vi "Get Pending IMatch Responses.vi"(8 "error in":errorcluster, 11 "Response Matcher in":refnum<class "Response Matcher.lvclass">) -> (0 "error out":errorcluster, 2 "Pending IMatch Responses":refnum<data-value>, 3 "Response Matcher out":refnum<class "Response Matcher.lvclass">)   [LabVIEW 2020, in "CANopen.lvlib" / "Response Matcher.lvlib" / "Response Matcher.lvclass"]
uses:
  Response Matcher.lvclass
  IResponse/IMatch Response.lvclass
  Response Matcher.lvclass/Response Matcher.ctl
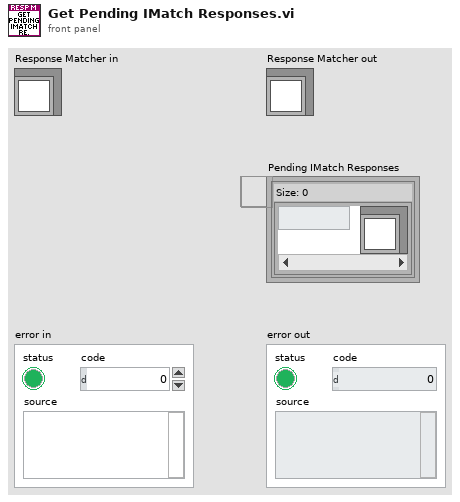
[diagram p1: front panel]
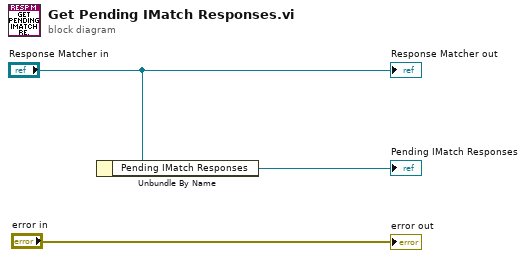
[diagram p0: block diagram]
diagram:
  n1 = Unbundle By Name("Response Matcher in") -> ("Pending IMatch Responses"=→"Pending IMatch Responses":refnum<data-value>)
  "error out" <- "error in"
  "Response Matcher out" <- "Response Matcher in"
